vi "Component Not Found.vi"(7 "error source vi name":string, 8 "error in (no error)":errorcluster, 10 "component name":string, 11 "Component Loader in":refnum<class "Component Loader.lvclass">) -> (0 "error out":errorcluster, 3 "Component Loader out":refnum<class "Component Loader.lvclass">)   [LabVIEW 2017, in "DSF Core.lvlib" / "Component Loader.lvclass"]
uses:
  Component Loader.lvclass
  Errors.ctl
  <vilib>/NI/Memory Manager/Static Error Handling.lvlib
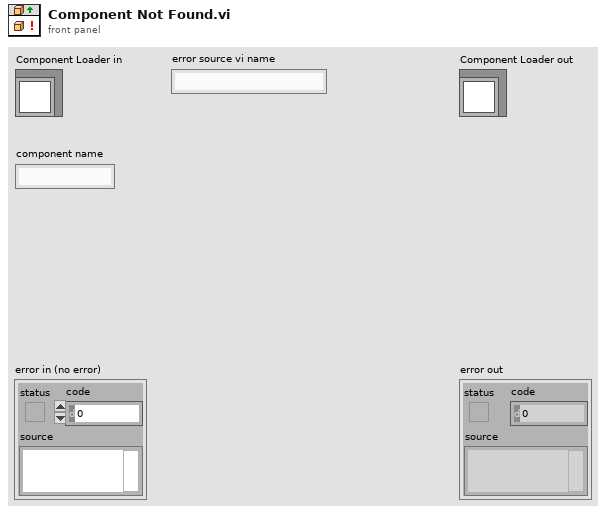
[diagram p1: front panel]
types:
  T1 = typedef "DSF Core.lvlib/Component Loader.lvclass/Errors.ctl" = enum16{"Component Directory Not Found", "Component Not Found", "Class Not Found"}
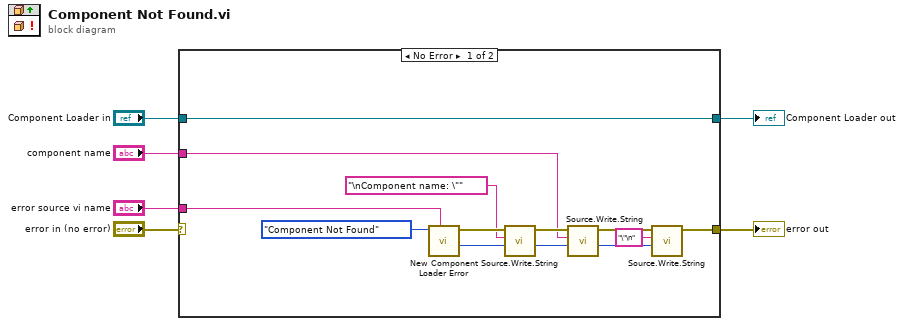
[diagram p0: block diagram]
diagram:
  n1 = case shown="No Error" "error in (no error)" {
    selector: "error in (no error)" -> [_ w21]
    tunnel: [w9 w21] -> w5
    tunnel: "error source vi name" -> [w18 _]
    tunnel: "Component Loader in" -> [w17 w20]
    tunnel: [w17 w20] -> w2
    tunnel: "component name" -> [w7 _]
    frame No Error {
      n2 = call "New Component Loader Error.vi"("error source vi name"=w18, "error"=Errors."Component Not Found") -> ("new offset"=w15:i32, "error out"=w16:errorcluster)  [unwired: 8 in]
      n3 = call <vilib>:"Source.Write.String.vi"("offset"=w15, "string"="\nComponent name: \"", "error in"=w16) -> ("new offset"=w14:i32, "error out"=w13:errorcluster)  [unwired: 7 in]
      n4 = call <vilib>:"Source.Write.String.vi"("offset"=w14, "string"=w7, "error in"=w13) -> ("new offset"=w10:i32, "error out"=w11:errorcluster)  [unwired: 7 in]
      n5 = call <vilib>:"Source.Write.String.vi"("offset"=w10, "string"="\"\n", "error in"=w11) -> ("error out"=w9:errorcluster)  [unwired: 7 in, 1 out]
    }
    frame Error {
    }
  }
  "error out" <- w5
  "Component Loader out" <- w2
